vi "ConfigTriggers.vi"(8 "error in (no error)":errorcluster, 11 "NiPxi6733 in":refnum<class "NiPxi6733.lvclass">) -> (0 "error out":errorcluster, 3 "NiPxi6733 out":refnum<class "NiPxi6733.lvclass">)   [LabVIEW 2018, in "FgenPlugins.lvlib" / "NiPxi6733.lvclass"]
uses:
  NiPxi6733.lvclass
  X:/Projects/NistPluggableModules/dev/NistPluggableModules/FGen/FgenPlugins/FgenPluginBaseClass/FgenPluginsBase.lvclass
  FgenPluginBaseClass/FgenPluginsBase.lvclass/FgenPluginsBase.ctl
  FgenPluginBaseClass/Read Triggers.vi
  FgenPluginBaseClass/Accessors/Read Channels.vi
  <vilib>/DAQmx/configure/trigger.llb/DAQmx Start Trigger (None).vi
  <vilib>/DAQmx/configure/trigger.llb/DAQmx Start Trigger (Digital Edge).vi
  <vilib>/Utility/error.llb/Error Cluster From Error Code.vi
  <vilib>/ErrorRing/Error Ring.xnode
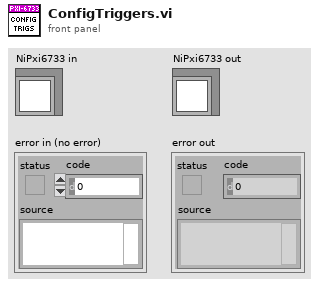
[diagram p1: front panel]
types:
  T1 = typedef "FgenPlugins.lvlib/Channel.ctl" = cluster{"Name":string, "Enabled":bool, "Operation":enum16{"Continuous", "Burst"}, "Impedance (50)":dbl, "Handle":string, "Connected":bool, "Mode (Function)":enum16{"Function", "Arbitrary", "Sequence"}}
  T2 = typedef "FgenPlugins.lvlib/clTriggers.ctl" = cluster{"Count":i32, "Triggers":T3[]}
  T3 = typedef "FgenPlugins.lvlib/Trigger.ctl" = cluster{"Source":string, "Slope":enum16{"Positive", "Negative", "Either"}, "Threshold":dbl, "Delay":dbl, "TriggerType":T4}
  T4 = typedef "FgenPlugins.lvlib/TriggerType.ctl" = enum16{"None", "Start", "Stop", "Hold", "Resume", "Advance"}
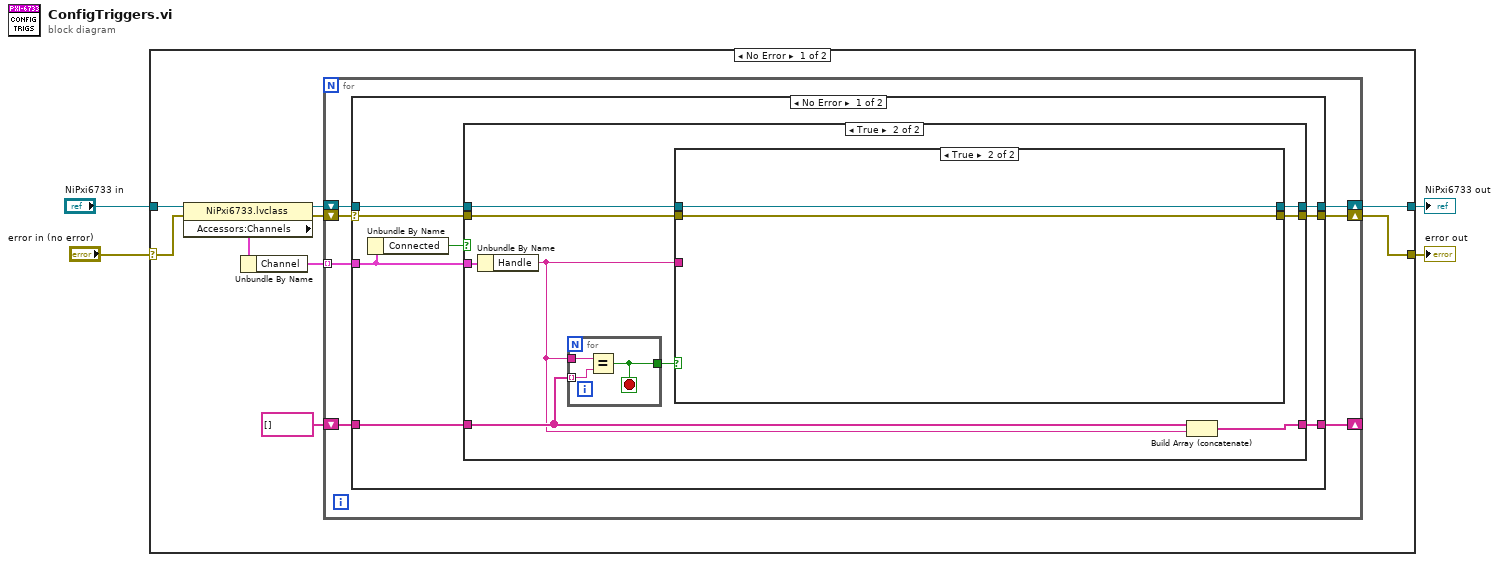
[diagram p0: block diagram]
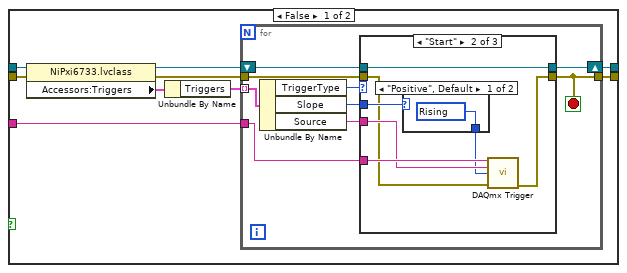
[diagram p3: hidden frame]
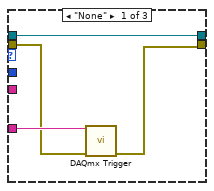
[diagram p4: hidden frame]
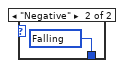
[diagram p5: hidden frame]
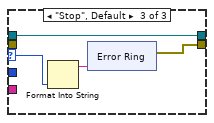
[diagram p6: hidden frame]
diagram:
  n1 = case shown="No Error" "error in (no error)" {
    selector: "error in (no error)" -> [w11 w91]
    tunnel: "NiPxi6733 in" -> [w13 w92]
    tunnel: [w5 w92] -> w2
    tunnel: [w6 w91] -> w1
    frame No Error {
      n2 = property class="NiPxi6733.lvclass"(reference=w13, error in=w11) -> (reference out=w12:refnum<class "NiPxi6733.lvclass">, error out=w10:errorcluster, "Accessors:Channels"=w9:cluster{"Count":u16, "Channel":T1[]})
      n3 = Unbundle By Name(w9) -> ("Channel"=w8:T1[])
      n4 = for {
        tunnel: w8 -> [w17] mode=indexing
        shift-right: [w16] -> _
        shift-left: string[] [] -> [w20]
        shift-right: [w14] -> w5
        shift-left: w12 -> [w19]
        shift-right: [w15] -> w6
        shift-left: w10 -> [w18]
        n5 = case shown="No Error" w18 {
          selector: w18 -> [w25 w89]
          tunnel: w20 -> [w27 w88]
          tunnel: w19 -> [w26 w90]
          tunnel: w17 -> [w24 _]
          tunnel: [w23 w88] -> w16
          tunnel: [w22 w89] -> w15
          tunnel: [w21 w90] -> w14
          frame No Error {
            n6 = Unbundle By Name(w24) -> ("Connected"=w28:bool)
            n7 = case shown="True" w28 {
              tunnel: w27 -> [w31 w38]
              tunnel: w26 -> [w29 w36]
              tunnel: w25 -> [w30 w35]
              tunnel: w24 -> [_ w40]
              tunnel: [w31 w39] -> w23
              tunnel: [w30 w34] -> w22
              tunnel: [w29 w32] -> w21
              frame False {
              }
              frame True {
                n8 = Unbundle By Name(w40) -> ("Handle"=w33:string)
                n9 = for {
                  tunnel: w38 -> [w86] mode=indexing
                  tunnel: w33 -> [w87]
                  tunnel: [w85] -> w37
                  stop <- w85 stop-if-true
                  n10 = Equal?(x=w87, y=w86) -> (x = y?=w85:bool)
                }
                n11 = case shown="True" w37 {
                  tunnel: w36 -> [w47 w84]
                  tunnel: [w42 w84] -> w32
                  tunnel: w35 -> [w48 w83]
                  tunnel: [w41 w83] -> w34
                  tunnel: w33 -> [w49 _]
                  frame False {
                    n12 = property class="NiPxi6733.lvclass"(reference=w47, error in=w48) -> (reference out=w43:refnum<class "NiPxi6733.lvclass">, error out=w44:errorcluster, "Accessors:Triggers"=w46:T2)
                    n13 = Unbundle By Name(w46) -> ("Triggers"=w45:T3[])
                    n14 = for {
                      tunnel: w49 -> [w58]
                      tunnel: w45 -> [w57] mode=indexing
                      tunnel: w44 -> [w54]
                      tunnel: [w52] -> w41
                      shift-right: [w53] -> w42
                      shift-left: w43 -> [w55]
                      stop <- w52 stop-if-true
                      n15 = Unbundle By Name(w57) -> ("TriggerType"=w56:T4, "Slope"=w51:enum16{"Positive", "Negative", "Either"}, "Source"=w50:string)
                      n16 = case shown="\"Start\"" w56 {
                        selector: w56 -> [_ _ w75]
                        tunnel: w58 -> [w62 w69 _]
                        tunnel: w55 -> [w60 w63 w73]
                        tunnel: w54 -> [w61 w65 _]
                        tunnel: [w60 w63 w73] -> w53
                        tunnel: [w59 w64 w72] -> w52
                        tunnel: w51 -> [_ w67 _]
                        tunnel: w50 -> [_ w68 _]
                        frame "None" {
                          n17 = call-poly <vilib>:"DAQmx Trigger.vi"("task/channels in"=w62, "error in"=w61) -> ("error out"=w59:errorcluster)  [unwired: 12 in, 1 out]
                        }
                        frame "Start" {
                          n18 = case shown="\"Positive\", Default" w67 {
                            tunnel: [w70 w71] -> w66
                            frame "Positive", Default {
                              w70 = 10280 items=["Rising"=10280, "Falling"=10171] ("edge")
                            }
                            frame "Negative" {
                              w71 = 10171 items=["Rising"=10280, "Falling"=10171] ("edge")
                            }
                          }
                          n19 = call-poly <vilib>:"DAQmx Trigger.vi"("task/channels in"=w69, "source"=w68, "edge"=w66, "error in"=w65) -> ("error out"=w64:errorcluster)  [unwired: 10 in, 1 out]
                        }
                        frame "Stop", Default {
                          n20 = Format Into String(w75) -> (resulting string=w74:string)  [unwired: 3 in, 1 out]
                          n21 = xnode "Error Ring"("parameter 0"=w74) -> ("error out"=w72:errorcluster)
                        }
                      }
                    }
                  }
                  frame True {
                  }
                }
                n22 = Build Array (concatenate)(w38, w33) -> (w39:string[])
              }
            }
          }
          frame Error {
          }
        }
      }
    }
    frame Error {
    }
  }
  "error out" <- w1
  "NiPxi6733 out" <- w2
